vi "Chronos TDMS Find Files for Date.vi"(8 "error in (no error)":errorcluster, 10 "time stamp":timestamp, 11 "path":path) -> (0 "error out":errorcluster, 2 "last file ID":i32, 3 "files":string[](array[string]))   [LabVIEW 2021]
uses:
  <vilib>/regexp/Match Regular Expression.xnode
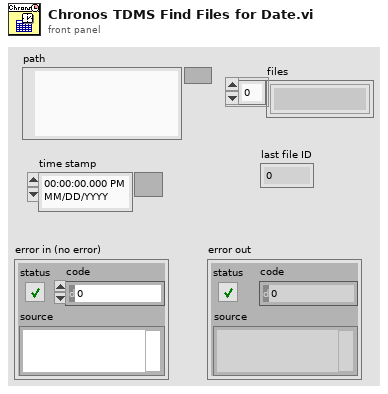
[diagram p1: front panel]
types:
  T1 = typedef "LVDateTimeRec.ctl" = cluster{"fractional second":dbl, "second":i32, "minute":i32, "hour":i32, "day of month":i32, "month":i32, "year":i32, "day of week":i32, "day of year":i32, "DST":i32}
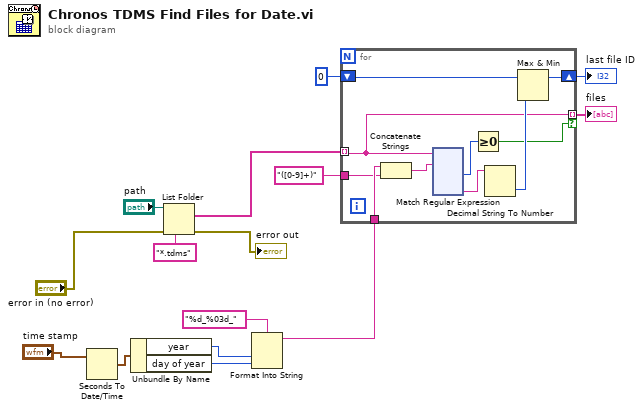
[diagram p0: block diagram]
diagram:
  n1 = Seconds To Date/Time(time stamp (now)="time stamp") -> (date time rec=w10:T1)  [unwired: 1 in]
  n2 = Unbundle By Name(w10) -> ("year"=w8:i32, "day of year"=w7:i32)
  n3 = List Folder(path="path", pattern="*.tdms", error in="error in (no error)") -> (filenames=w14:string[], error out=→"error out":errorcluster)  [unwired: 1 in, 2 out]
  n4 = Format Into String(format string="%d_%03d_", w8, w7) -> (resulting string=w5:string)  [unwired: 2 in, 1 out]
  n5 = for {
    tunnel: w14 -> [w18] mode=indexing
    tunnel: w5 -> [w25]
    tunnel: "([0-9]+)" -> [w24]
    shift-right: [w19] -> w4
    shift-left: 0 -> [w20]
    tunnel: [w18] -> w3 mode=indexing if=w16
    n6 = Concatenate Strings(w25, w24) -> (w23:string)
    n7 = xnode "Match Regular Expression"("input string"=w18, "regular expression"=w23) -> ("offset past match"=w17:i32, "submatch 1"=w22:string)  [unwired: 4 in, 4 out]
    n8 = Greater Or Equal To 0?(x=w17) -> (x >= 0?=w16:bool)
    n9 = Decimal String To Number(string=w22) -> (number=w21:i32)  [unwired: 2 in, 1 out]
    n10 = Max & Min(x=w20, y=w21) -> (max(x,y)=w19:i32)  [unwired: 1 out]
  }
  "last file ID" <- w4
  "files" <- w3
